vi "Parse Bits.vi"(8 "error in (no error)":errorcluster, 11 "Literal in":refnum<class "Literal.lvclass">) -> (0 "error out":errorcluster, 3 "Literal out":refnum<class "Literal.lvclass">)   [LabVIEW 2020, in "Literal.lvclass"]
uses:
  Literal.lvclass
  C:/dev/IlluminatedG/AdventOfCode/2021/source/Day 16/Part 1/Packet/Packet.lvclass
  Literal.lvclass/Literal.ctl
  Packet/Packet.lvclass
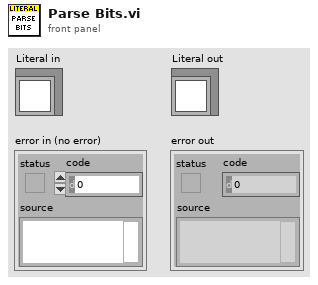
[diagram p1: front panel]
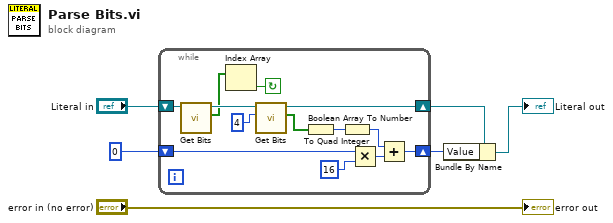
[diagram p0: block diagram]
diagram:
  n1 = while {
    shift-right: [w16] -> w3
    shift-left: i64 0 -> [w19]
    shift-right: [w7] -> w4
    shift-left: "Literal in" -> [w15]
    stop <- w11 continue-if-true
    n2 = call "Get Bits.vi"("Packet in"=w15) -> ("Bits"=w12:bool[], "Packet out"=w14:refnum<class "Literal.lvclass">)  [unwired: 8 in, 1 out]
    n3 = Index Array(array=w12) -> (element=w11:bool)  [unwired: 1 in]
    n4 = call "Get Bits.vi"("Count (1)"=4, "Packet in"=w14) -> ("Bits"=w10:bool[], "Packet out"=w7:refnum<class "Literal.lvclass">)  [unwired: 7 in, 1 out]
    n5 = Boolean Array To Number(Boolean array=w10) -> (number=w9:u32)
    n6 = To Quad Integer(1:w9) -> (0:w8:i64)
    n7 = Multiply(x=w19, y=i64 16) -> (x*y=w17:i64)
    n8 = Add(x=w8, y=w17) -> (x+y=w16:i64)
  }
  n9 = Bundle By Name(cluster=w4, "Value"=w3) -> (→"Literal out":refnum<class "Literal.lvclass">)
  "error out" <- "error in (no error)"
